vi "Example Test 1.vi"(5 "b 2":dbl=4.0, 7 "a 2":dbl=3.0, 8 "error in (no error)":errorcluster, 9 "string control try":string, 11 "a":dbl=1.0) -> (0 "error out":errorcluster, 1 "myString":string, 2 "signal out 2":waveform(dbl), 3 "signal out":waveform(dbl), 4 "output A3 double":dbl=3.0)   [LabVIEW 2014]
doc: "This VI is created for purpose of testing transcriptor. It Contains two WhileLoop with some constants inside, just to verify if it's possible to parse VI and got some relevant info."
uses:
  <vilib>/measure/NI_MABase.lvlib
panel:
  out "x+y 2":i16
  out "x+y":i32
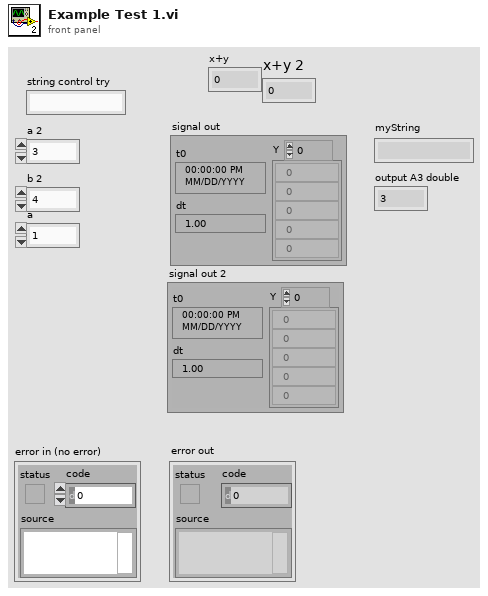
[diagram p1: front panel]
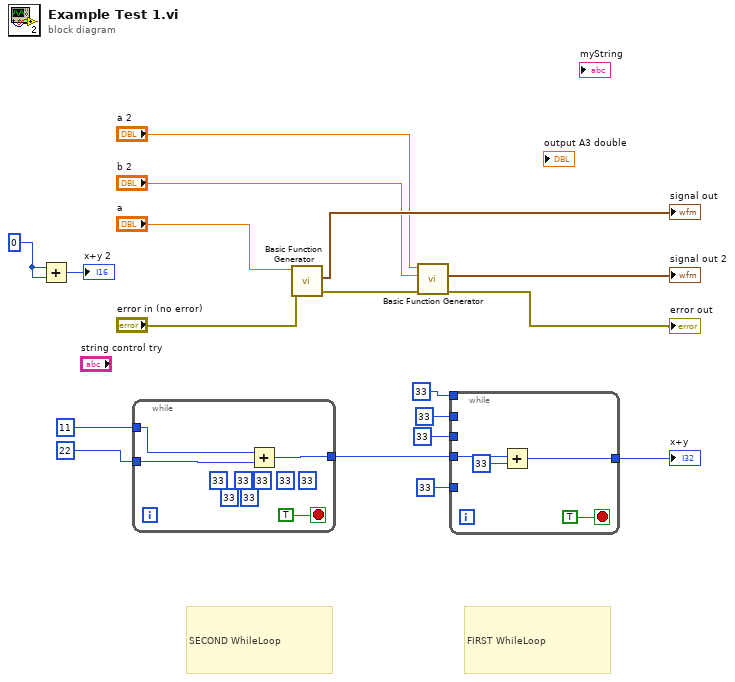
[diagram p0: block diagram]
diagram:
  w1 = i16 0 ("y")
  # "SECOND WhileLoop"
  # "FIRST WhileLoop"
  n1 = Add(x=w1, y=w1) -> (x+y=→"x+y 2":i16)
  n2 = while {
    tunnel: 11 ("Numeric") -> [w21]
    tunnel: 22 ("Numeric 2") -> [w20]
    tunnel: [w19] -> w8
    stop <- TRUE stop-if-true
    (unwired) 33 ("y")
    (unwired) 33 ("y")
    (unwired) 33 ("y")
    (unwired) 33 ("y")
    (unwired) 33 ("y")
    (unwired) 33 ("y")
    (unwired) 33 ("y")
    n3 = Add(x=w21, y=w20) -> (x+y=w19:i32)
  }
  n4 = call <vilib>:"Basic Function Generator.vi"("error in (no error)"="error in (no error)", "frequency"="a") -> ("error out"=w15:errorcluster, "signal out"=→"signal out":waveform(dbl))  [unwired: 7 in, 1 out]
  n5 = call <vilib>:"Basic Function Generator.vi"("error in (no error)"=w15, "amplitude"="b 2", "frequency"="a 2") -> ("error out"=→"error out":errorcluster, "signal out"=→"signal out 2":waveform(dbl))  [unwired: 6 in, 1 out]
  n6 = while {
    tunnel: w8 -> [w25]
    tunnel: [w23] -> w7
    tunnel: 33 ("y") -> [_]
    tunnel: 33 ("y") -> [_]
    tunnel: 33 ("y") -> [_]
    tunnel: 33 ("y") -> [_]
    stop <- TRUE stop-if-true
    n7 = Add(x=w25, y=33) -> (x+y=w23:i32)
  }
  "x+y" <- w7
